vi "Get Magnet.vi"(6 "Axis":T1=enum."Z", 8 "error in (no error)":errorcluster, 11 "Instrument.Oxford1820 in":refnum<class "Instrument.Oxford1820.lvclass">) -> (0 "error out":errorcluster, 1 "Status":string, 2 "B Field (T)":dbl, 3 "Instrument.Oxford1820 out":refnum<class "Instrument.Oxford1820.lvclass">, 4 "Finished?":bool)   [LabVIEW 2019, in "Instrument.Oxford1820.lvclass"]
uses:
  Instrument.Oxford1820.lvclass
  <userlib>/LevyLab/Instrument Framework/Instrument Types/Cryostat/Typedefs/Magnet Axis--Enum.ctl
  d637c3ba-c61f-4734-ba3b-69dfccbf1047.vi/3b273696-eb05-4b68-bbc6-50a3f139d26e.vi
  d637c3ba-c61f-4734-ba3b-69dfccbf1047.vi/24f4d168-9f7f-4813-a6b1-dc4d2581702a.vi
  <vilib>/Utility/Data Type/Get Type Information.vi
  <vilib>/JDP Science/JSONtext/JSON text to Variant.vi
  <vilib>/JDP Science/JSONtext/LVClass Serializer/JSONtext LVClass Serializer.lvclass
  <userlib>/LevyLab/Instrument Framework/Instrument Types/Cryostat/Instrument.Cryostat.lvclass
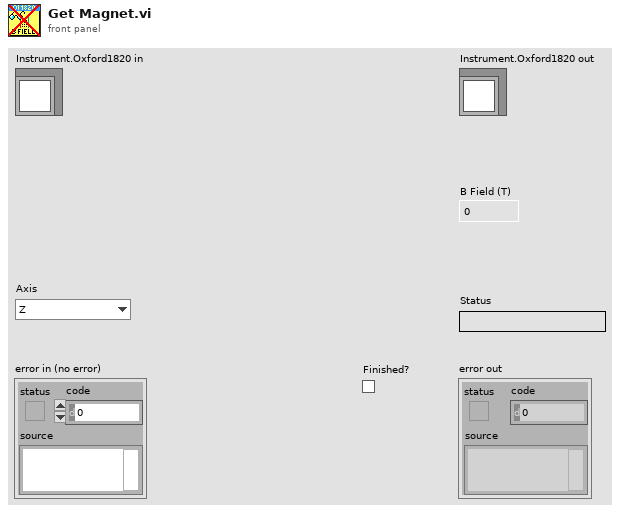
[diagram p1: front panel]
types:
  T1 = typedef "Instrument.Cryostat.lvclass/Magnet Axis--Enum.ctl" = enum16{"X", "Y", "Z"}
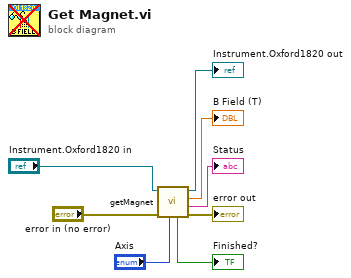
[diagram p0: block diagram]
diagram:
  n1 = call-dynamic "getMagnet.vi"("Axis"="Axis", "error in (no error)"="error in (no error)", "Instrument.Oxford1820 in"="Instrument.Oxford1820 in") -> ("error out"=→"error out":errorcluster, "Status"=→"Status":string, "B Field (T)"=→"B Field (T)":dbl, "Instrument.Oxford1820 out"=→"Instrument.Oxford1820 out":refnum<class "Instrument.Oxford1820.lvclass">, "Finished?"=→"Finished?":bool)  [unwired: 4 in]
